vi "Send onNotification.vi"(8 "error in (no error)":errorcluster, 10 "request":string, 11 "id":i32) -> (0 "error out":errorcluster)   [LabVIEW 2025, in "MCP Server.lvlib"]
uses:
  MCP Server.lvlib
  onNotification.ctl
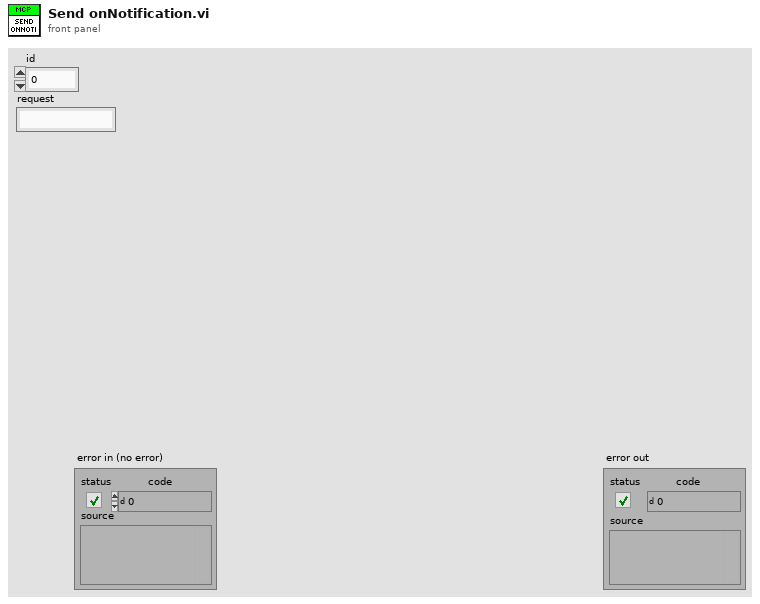
[diagram p1: front panel]
types:
  T1 = typedef "MCP Server.lvlib/onNotification.ctl" = cluster{"request":string}
  T2 = typedef "MCP Server.lvlib/Server Data.ctl" = cluster{"Name":string, "Description":string, "Tools":T3[], "Parameters":string[][], "Logging Info":T6, "User Events":T7}
  T3 = typedef "MCP Server.lvlib/Tool Data.ctl" = cluster{"Name":string, "Description":string, "Ignored":string[], "VI path":path, "inputs":T4[], "outputs":T5[]}
  T4 = typedef "MCP Server.lvlib/Input Parameter.ctl" = cluster{"name":string, "type":string, "description":string, "required":bool, "raw name":string}
  T5 = typedef "MCP Server.lvlib/Output Parameter.ctl" = cluster{"name":string, "description":string, "type":string, "raw name":string}
  T6 = typedef "MCP Server.lvlib/Logging.ctl" = cluster{"Log":string[], "Max Length":i32}
  T7 = typedef "MCP Server.lvlib/User Events.ctl" = cluster{"onError":refnum<user-event>, "onLog":refnum<user-event>, "onConnect":refnum<user-event>, "onToolsList":refnum<user-event>, "onToolsCall":refnum<user-event>, "onNotification":refnum<user-event>, "onTool":refnum<user-event>, "onRpc":refnum<user-event>}
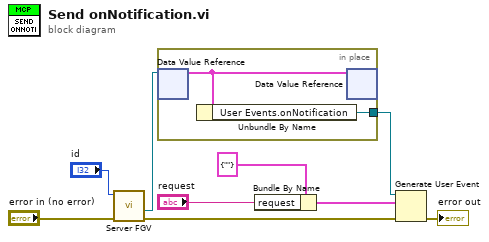
[diagram p0: block diagram]
diagram:
  n1 = call "Server FGV.vi"("error in"="error in (no error)", "id"="id") -> ("error in 2"=w8:errorcluster, "server reference"=w5:refnum<data-value>)  [unwired: 5 in, 3 out]
  n2 = in-place {
    in-place-border: [w10] -> w4
    n3 = in-place-dvr #1(w5) -> (w11:T2)  [unwired: 1 out]
    n4 = Unbundle By Name(w11) -> ("User Events.onNotification"=w10:refnum<user-event>)
    n5 = in-place-dvr #1(w11) -> ()  [unwired: 2 out]
  }
  n6 = Bundle By Name(cluster=T1 {"request"=""} ("event data"), "request"="request") -> (w2:T1)
  n7 = Generate User Event(user event=w4, event data cluster=w2, error in=w8) -> (error out=→"error out":errorcluster)  [unwired: 1 in, 1 out]
